vi "Actor Core.vi"(8 "error in":errorcluster, 11 "TDMS Data Source in":refnum<class "TDMS Data Source.lvclass">) -> (0 "error out":errorcluster, 3 "Actor out":refnum<class "Actor.lvclass">)   [LabVIEW 2020, in "TDMS Data Source.lvlib" / "TDMS Data Source.lvclass"]
doc: "<p>(<strong>Filename</strong>: <span class=\"dnl\">Actor Framework.lvlib:Actor.lvclass:Actor Core.vi</span>)</p>\n<p>Receives messages to the actor, reacts to them, and initiates any error handling that may shut the actor down.</p>\n<p>Descendant classes may override this VI to append parallel tasks for the actor to complete while it handles messages. Overrides use the <a href=\"nihelplauncher://docs/csh?context=lvcore_glang_udclass\">Call Parent Class Method</a> node.</p>"
uses:
  TDMS Data Source.lvclass
  C:/Program Files/National Instruments/LabVIEW 2026/vi.lib/ActorFramework/Actor/Actor.lvclass
  <vilib>/ActorFramework/Actor/Actor.lvclass
  QMH Message.ctl
  TDMS Data Source.lvclass/TDMS Data Source.ctl
  <vilib>/ActorFramework/Actor/Actor.lvclass/Actor.ctl
  <vilib>/ActorFramework/Message Enqueuer/Message Enqueuer.lvclass/Message Enqueuer.ctl
  TDMS Data Source Messages/Done Reading File Msg/Done Reading File Msg.lvclass/Done Reading File Msg.ctl
  Application Manager/Application Manager Messages/Broadcast Data Source Info String Msg/Broadcast Data Source Info String Msg.lvclass/Broadcast Data Source Info String Msg.ctl
  <vilib>/ActorFramework/Message Enqueuer/Init from Existing Queue.vi
  <vilib>/ActorFramework/Message Enqueuer/Enqueue.vi
  TDMS Data Source Messages/Done Reading File Msg/Done Reading File Msg.lvclass
  C:/Program Files/National Instruments/LabVIEW 2026/vi.lib/ActorFramework/Message/Message.lvclass
  Application Manager/Application Manager Messages/Broadcast Data Source Info String Msg/Broadcast Data Source Info String Msg.lvclass
  <vilib>/ActorFramework/Message Priority Queue/Priority Enqueue.vi
  Data Source/Data Source/Data Source.lvclass
  <vilib>/ActorFramework/Message Enqueuer/Message Enqueuer.lvclass
panel:
  out "Debug: Allocation Speed":dbl(graph)
  out "Debug: Read Speed":waveform(dbl)(graph)
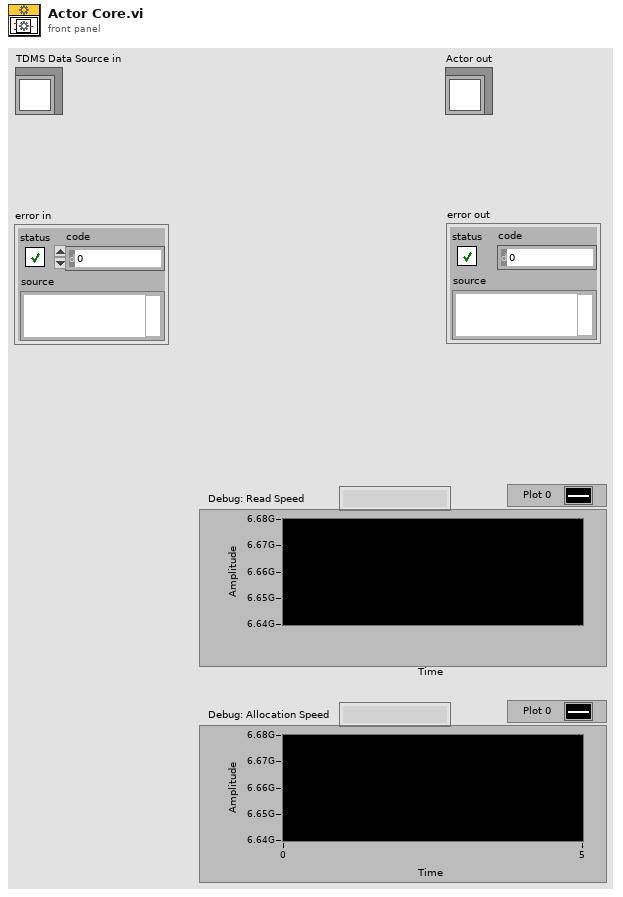
[diagram p1: front panel]
types:
  T1 = typedef "TDMS Data Source.lvlib/TDMS Data Source.lvclass/QMH Message.ctl" = cluster{"Command":string, "Data":variant}
  T2 = enum16{"open", "open or create", "create or replace", "create", "open (read-only)"}
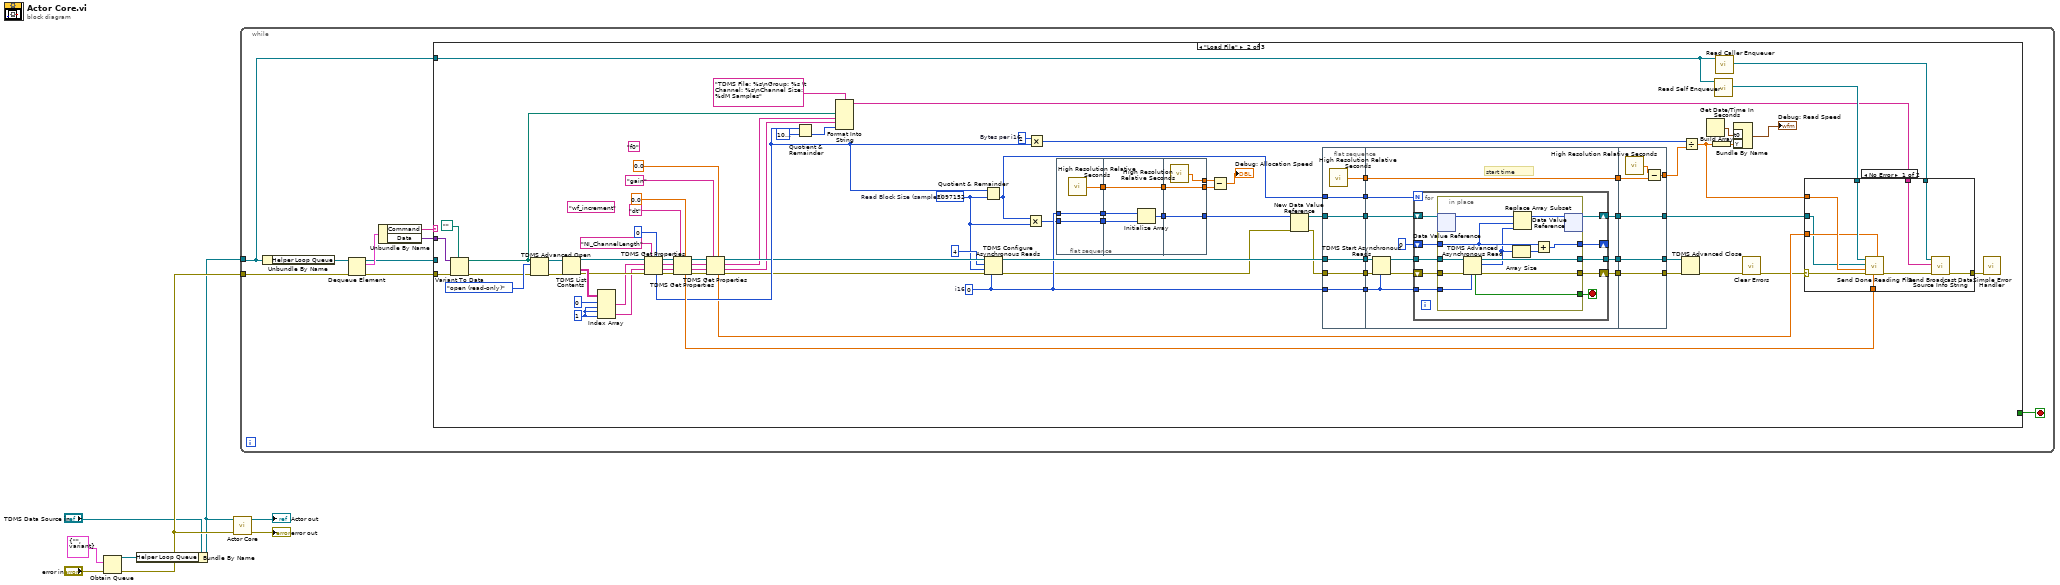
[diagram p0: block diagram]
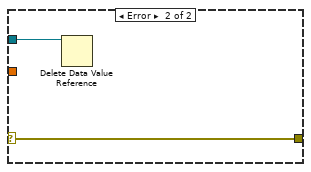
[diagram p3: hidden frame]
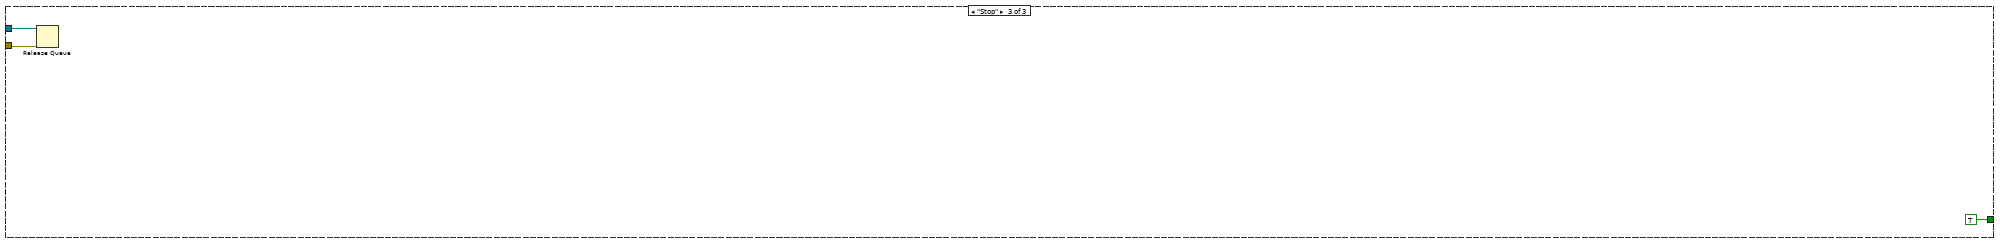
[diagram p4: hidden frame]
diagram:
  n1 = Obtain Queue(element data type=T1 {"Command"="", "Data"=variant}, error in (no error)="error in") -> (queue out=w3:refnum<queue>, error out=w4:errorcluster)  [unwired: 3 in, 1 out]
  n2 = Bundle By Name(cluster="TDMS Data Source in", "Helper Loop Queue"=w3) -> (w1:refnum<class "TDMS Data Source.lvclass">)
  n3 = call-parent "Actor Core.vi"("error in"=w4, "Actor in"=w1) -> ("error out"=→"error out":errorcluster, "Actor out"=→"Actor out":refnum<class "Actor.lvclass">)  [unwired: 8 in]
  n4 = while {
    tunnel: w4 -> [w17]
    tunnel: w1 -> [w10]
    stop <- w11 stop-if-true
    n5 = Unbundle By Name(w10) -> ("Helper Loop Queue"=w9:refnum<queue>)
    n6 = Dequeue Element(queue=w9, error in (no error)=w17) -> (queue out=w14:refnum<queue>, element=w16:T1, error out=w13:errorcluster)  [unwired: 1 in, 1 out]
    n7 = Unbundle By Name(w16) -> ("Command"=w15:string, "Data"=w12:variant)
    n8 = case shown="\"Load File\"" w15 {
      tunnel: w14 -> [_ _ w172]
      tunnel: w13 -> [_ w100 w171]
      tunnel: w12 -> [_ w101 _]
      tunnel: [_ _ TRUE] -> w11
      tunnel: w10 -> [_ w74 _]
      frame Default {
      }
      frame "Load File" {
        (unwired) "f0" ("property name")
        w20 = u64 2097152  # Read Block Size (samples)
        w34 = u64 2  # Bytes per i16
        w31 = i16 0  # i16
        (unwired) "wf_increment" ("property name")
        w95 = 1 ("disabled index (col)")
        n9 = Variant To Data(error in=w100, type=path "" ("appended path"), Variant=w101) -> (data=w71:path, error out=w86:errorcluster)
        n10 = TDMS Advanced Open(8:w86, 10:T2."open (read-only)" ("Operation"), 11:w71) -> (0:w88:errorcluster, 3:w87:refnum<k34>)  [unwired: 2 in, 1 out]
        n11 = TDMS List Contents(4:w88, 7:w87) -> (0:w94:errorcluster, 1:w97:string[][], 3:w93:refnum<k34>)  [unwired: 1 in, 1 out]
        n12 = Index Array(array=w97, index (row) #1=0 ("index (row)"), index (col) #1=w95, index (row) #2=w95, index (col) #2=w95) -> (element #1=w92:string, element #2=w91:string)
        n13 = TDMS Get Properties(5:u32 0, 7:"NI_ChannelLength" ("property name"), 8:w94, 9:w91, 10:w92, 11:w93) -> (0:w78:errorcluster, 1:w69:string, 2:w70:string, 3:w79:refnum<k34>, 4:w67:u32)  [unwired: 1 out]
        n14 = TDMS Get Properties(5:0.0, 7:"dt" ("property name"), 8:w78, 9:w69, 10:w70, 11:w79) -> (0:w63:errorcluster, 1:w59:string, 2:w60:string, 3:w64:refnum<k34>, 4:w75:dbl)  [unwired: 1 out]
        n15 = TDMS Get Properties(5:0.0, 7:"gain" ("property name"), 8:w63, 9:w59, 10:w60, 11:w64) -> (0:w61:errorcluster, 1:w57:string, 2:w58:string, 3:w62:refnum<k34>, 4:w54:dbl)  [unwired: 1 out]
        n16 = Quotient & Remainder(x=w67, y=u32 1000000) -> (floor(x/y)=w66:u32)  [unwired: 1 out]
        n17 = Format Into String(format string="TDMS File: %s\nGroup: %s \t Channel: %s\nChannel Size: %dM Samples", w71, w58, w57, w66) -> (resulting string=w68:string)  [unwired: 2 in, 1 out]
        n18 = Quotient & Remainder(x=w67, y=w20) -> (floor(x/y)=w24:u64)  [unwired: 1 out]
        n19 = TDMS Configure Asynchronous Reads(6:w31, 8:w61, 9:w20, 10:u32 4 ("number of buffers (4)"), 11:w62) -> (0:w23:errorcluster, 3:w35:refnum<k34>)  [unwired: 1 in]
        n20 = Multiply(x=w24, y=w20) -> (x*y=w21:u64)
        n21 = Multiply(x=w34, y=w67) -> (x*y=w32:u64)
        n22 = flat-sequence {
          tunnel: w31 -> [w104]
          tunnel: [w104] -> w42
          tunnel: [w103] -> w41
          tunnel: w21 -> [w103]
          tunnel: [w102] -> w40
          tunnel: [w108] -> w39
          tunnel: w42 -> [w106]
          tunnel: w41 -> [w105]
          tunnel: [w107] -> w38
          tunnel: w40 -> [w107]
          tunnel: [w111] -> w30
          tunnel: w39 -> [w111]
          tunnel: [w110] -> w27
          tunnel: [w109] -> w25
          tunnel: w38 -> [w109]
          frame #0 {
            n23 = call <vilib>:"High Resolution Relative Seconds.vi"() -> ("relative seconds"=w102:dbl)
          }
          frame #1 {
            n24 = Initialize Array(w106, w105) -> (w108:i16[])
          }
          frame #2 {
            n25 = call <vilib>:"High Resolution Relative Seconds.vi"() -> ("relative seconds"=w110:dbl)
          }
        }
        n26 = Subtract(x=w27, y=w25) -> (x-y=→"Debug: Allocation Speed":dbl)
        n27 = New Data Value Reference(data value=w30, error in=w23) -> (data value reference=w29:refnum<data-value>, error out=w28:errorcluster)
        n28 = flat-sequence {
          tunnel: w28 -> [w117]
          tunnel: [w117] -> w52
          tunnel: w35 -> [w116]
          tunnel: [w116] -> w51
          tunnel: [w115] -> w50
          tunnel: [w114] -> w49
          tunnel: w24 -> [w114]
          tunnel: [w113] -> w48
          tunnel: w31 -> [w113]
          tunnel: [w112] -> w47
          tunnel: w29 -> [w112]
          tunnel: w52 -> [w123]
          tunnel: w51 -> [w122]
          tunnel: w50 -> [w129]
          tunnel: [w129] -> w46
          tunnel: [w128] -> w45
          tunnel: [w127] -> w44
          tunnel: w49 -> [w126]
          tunnel: w48 -> [w119]
          tunnel: w47 -> [w125]
          tunnel: [w124] -> w43
          tunnel: w46 -> [w156]
          tunnel: w45 -> [w155]
          tunnel: [w155] -> w37
          tunnel: [w154] -> w36
          tunnel: w44 -> [w154]
          tunnel: [w153] -> w33
          tunnel: [w152] -> w19
          tunnel: w43 -> [w152]
          frame #0 {
            n29 = call <vilib>:"High Resolution Relative Seconds.vi"() -> ("relative seconds"=w115:dbl)
          }
          frame #1 {
            # "start time"
            n30 = TDMS Start Asynchronous Reads(6:w119, 8:w123, 11:w122) -> (0:w120:errorcluster, 3:w121:refnum<k34>)  [unwired: 1 in]
            n31 = for {
              N: w126 -> [_]
              tunnel: [w134] -> w128
              shift-right: [w139] -> w127
              shift-left: w120 -> [w136]
              tunnel: w121 -> [w135]
              tunnel: w119 -> [w137]
              shift-right: [w133] -> w124
              shift-left: w125 -> [w138]
              shift-right: [w130] -> _
              shift-left: 0 -> [w131]
              stop <- w132 stop-if-true
              n32 = in-place {
                in-place-border: [w147] -> w139
                in-place-border: w137 -> [w150]
                in-place-border: w136 -> [w149]
                in-place-border: w135 -> [w148]
                in-place-border: [w146] -> w134
                in-place-border: [w145] -> w132
                in-place-border: w131 -> [w144]
                in-place-border: [w142] -> w130
                n33 = in-place-dvr #1(w138) -> (w151:i16[])  [unwired: 1 out]
                n34 = TDMS Advanced Asynchronous Read(6:w150, 8:w149, 11:w148) -> (0:w147:errorcluster, 2:w140:i16[], 3:w146:refnum<k34>, 4:w145:bool)
                n35 = Array Size(array=w140) -> (size(s)=w143:i32)
                n36 = Replace Array Subset(array=w151, new element=w140, index=w144) -> (w141:i16[])
                n37 = Add(x=w144, y=w143) -> (x+y=w142:i32)
                n38 = in-place-dvr #1(w141) -> (w133:refnum<data-value>)  [unwired: 1 out]
              }
            }
          }
          frame #2 {
            n39 = call <vilib>:"High Resolution Relative Seconds.vi"() -> ("relative seconds"=w157:dbl)
            n40 = Subtract(x=w157, y=w156) -> (x-y=w153:dbl)
          }
        }
        n41 = TDMS Advanced Close(8:w36, 11:w37) -> (0:w53:errorcluster)  [unwired: 2 in, 1 out]
        n42 = Divide(x=w32, y=w33) -> (x/y=w80:dbl)
        n43 = Get Date/Time In Seconds() -> (seconds since 1Jan1904=w83:timestamp)
        n44 = Build Array(w80) -> (w84:dbl[])
        n45 = call <vilib>:"Read Self Enqueuer.vi"("Actor"=w74) -> ("Self Enqueuer"=w82:refnum<class "Message Enqueuer.lvclass">)  [unwired: 10 in]
        n46 = call <vilib>:"Read Caller Enqueuer.vi"("Actor"=w74) -> ("Caller Enqueuer"=w73:refnum<class "Message Enqueuer.lvclass">)  [unwired: 10 in]
        n47 = Bundle By Name("t0"=w83, "Y"=w84) -> (→"Debug: Read Speed":waveform(dbl))  [unwired: 1 in]
        n48 = call <vilib>:"Clear Errors.vi"("error in (no error)"=w53) -> ("error out"=w18:errorcluster)  [unwired: 5 in, 1 out]
        n49 = case shown="No Error" w18 {
          selector: w18 -> [w167 w169]
          tunnel: w82 -> [w166 _]
          tunnel: [w162 w169] -> w81
          tunnel: w80 -> [w164 _]
          tunnel: w75 -> [w163 _]
          tunnel: w73 -> [w161 _]
          tunnel: w68 -> [w160 _]
          tunnel: w54 -> [w159 _]
          tunnel: w19 -> [w158 w168]
          frame No Error {
            n50 = call "Send Done Reading File.vi"("gain"=w159, "dt"=w163, "error in (no error)"=w167, "Read Speed"=w164, "Data Buffer"=w158, "Message Enqueuer"=w166) -> ("error out"=w165:errorcluster)  [unwired: 4 in, 1 out]
            n51 = call "Send Broadcast Data Source Info String.vi"("error in (no error)"=w165, "Data Source Info String"=w160, "Message Enqueuer"=w161) -> ("error out"=w162:errorcluster)  [unwired: 7 in, 1 out]
          }
          frame Error {
            n52 = Delete Data Value Reference(data value reference=w168) -> ()  [unwired: 1 in, 2 out]
          }
        }
        n53 = call <vilib>:"Simple Error Handler.vi"("error in (no error)"=w81) -> ()  [unwired: 1 in, 8 out]
      }
      frame "Stop" {
        n54 = Release Queue(queue=w172, error in (no error)=w171) -> ()  [unwired: 1 in, 3 out]
      }
    }
  }
